vi "Init Static.vi"(8 "error in (no error)":errorcluster, 9 "Caller Queue":refnum<class "Priority Message Queue.lvclass">, 10 "Self Queue":refnum<class "Priority Message Queue.lvclass">, 11 "Actor API in":refnum<class "Actor API.lvclass">) -> (0 "error out":errorcluster, 3 "Actor API out":refnum<class "Actor API.lvclass">)   [LabVIEW 2022 SP3, in "Artifex.lvlib" / "Actor API.lvclass"]
uses:
  Actor API.lvclass
  Actor API.lvclass/Actor API.ctl
  Priority Message Queue/Priority Message Queue.lvclass
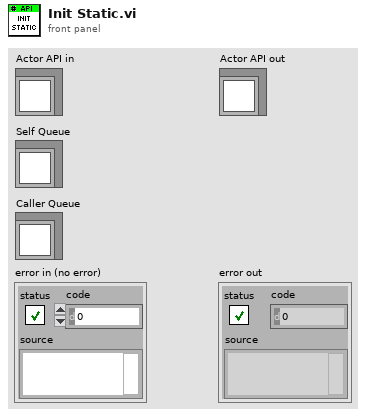
[diagram p1: front panel]
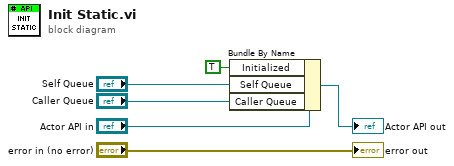
[diagram p0: block diagram]
diagram:
  n1 = Bundle By Name(cluster="Actor API in", "Initialized"=TRUE, "Self Queue"="Self Queue", "Caller Queue"="Caller Queue") -> (→"Actor API out":refnum<class "Actor API.lvclass">)
  "error out" <- "error in (no error)"
